vi "master_panel.vi"() -> ()   [LabVIEW 2015]
panel:
  out "Genotype":string
  out "Timestamp":string
  out "Fly Name":string
  out "Experiment Name":string
  in  "Metadata Path":path
  in  "Randomize":bool
  in  "Protocol Path":path
  out "Protocol Name":path
  out "Experiment Path":path
  in  "N Reps":dbl
  in  "Use Test File":bool
  in  "New Rec":bool
  in  "Experiment Session Control":enum32{"recording", "roi"}(radio)
  in  "run_protocol":bool
  in  "open_stimulus":bool
  in  "open_physiology":bool
  in  "open_imaging":bool
  in  "exit_button":bool
  # "Metadata"
  # "Protocol"
  # "Control Panels"
  # "Recording"
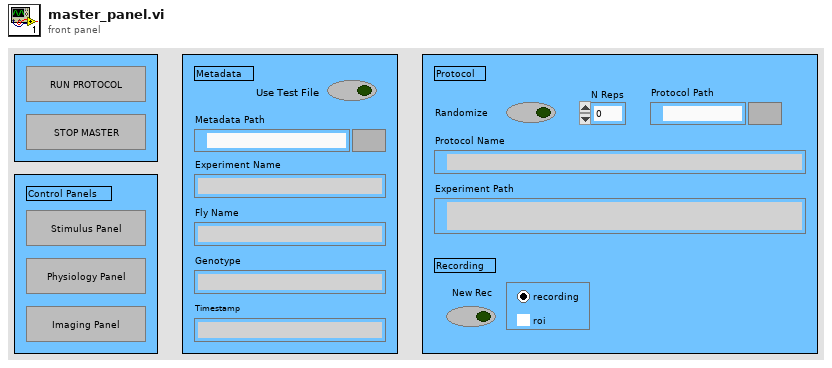
[diagram p1: front panel]
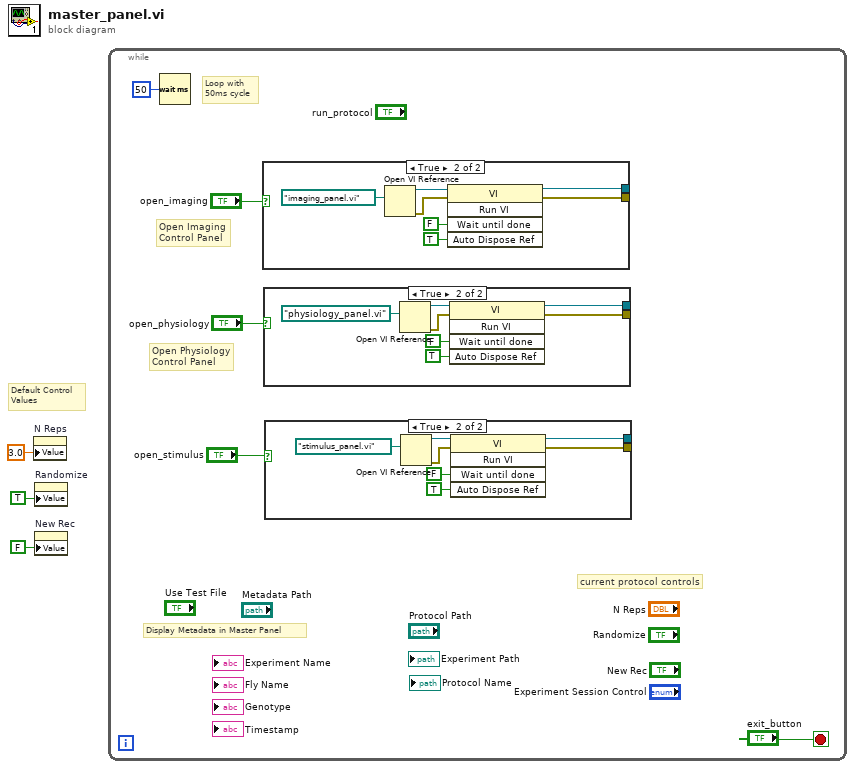
[diagram p0: block diagram]
diagram:
  # "Default Control\nValues"
  n1 = property on="N Reps" class="DigNum (strict)"("Value"=3.0 ("N Reps")) -> ()  [unwired: 2 in, 2 out]
  n2 = property on="Randomize" class="Bool (strict)"("Value"=TRUE ("Randomize")) -> ()  [unwired: 2 in, 2 out]
  n3 = property on="New Rec" class="Bool (strict)"("Value"=FALSE ("New Rec")) -> ()  [unwired: 2 in, 2 out]
  n4 = while {
    stop <- "exit_button" stop-if-true
    # "current protocol controls"
    # "Display Metadata in Master Panel"
    # "Open Physiology\nControl Panel"
    # "Open Imaging \nControl Panel"
    # "Loop with\n50ms cycle"
    n5 = Wait (ms)(milliseconds to wait=u32 50) -> ()  [unwired: 1 out]
    n6 = case shown="True" "open_imaging" {
      tunnel: [_ w24] -> _
      tunnel: [_ w23] -> _
      frame False {
      }
      frame True {
        n7 = Open VI Reference(vi path=path "imaging_panel.vi") -> (vi reference=w28:refnum<vi>, error out=w27:errorcluster)  [unwired: 5 in]
        n8 = invoke class="VI" method="Run VI"(reference=w28, error in=w27, "Wait until done"=FALSE ("Wait Until Done"), "Auto Dispose Ref"=TRUE ("Auto Dispose Reference")) -> (reference out=w24:refnum<vi>, error out=w23:errorcluster)  [unwired: 1 in, 3 out]
      }
    }
    n9 = case shown="True" "open_physiology" {
      tunnel: [_ w17] -> _
      tunnel: [_ w16] -> _
      frame False {
      }
      frame True {
        n10 = Open VI Reference(vi path=path "physiology_panel.vi") -> (vi reference=w21:refnum<vi>, error out=w20:errorcluster)  [unwired: 5 in]
        n11 = invoke class="VI" method="Run VI"(reference=w21, error in=w20, "Wait until done"=FALSE ("Wait Until Done"), "Auto Dispose Ref"=TRUE ("Auto Dispose Reference")) -> (reference out=w17:refnum<vi>, error out=w16:errorcluster)  [unwired: 1 in, 3 out]
      }
    }
    n12 = case shown="True" "open_stimulus" {
      tunnel: [_ w10] -> _
      tunnel: [_ w9] -> _
      frame False {
      }
      frame True {
        n13 = Open VI Reference(vi path=path "stimulus_panel.vi") -> (vi reference=w14:refnum<vi>, error out=w13:errorcluster)  [unwired: 5 in]
        n14 = invoke class="VI" method="Run VI"(reference=w14, error in=w13, "Wait until done"=FALSE ("Wait Until Done"), "Auto Dispose Ref"=TRUE ("Auto Dispose Reference")) -> (reference out=w10:refnum<vi>, error out=w9:errorcluster)  [unwired: 1 in, 3 out]
      }
    }
  }
